vi "Generate Window Name.vi"(10 "Module Name":string, 11 "Item Name":string) -> (3 "Window Name":string)   [LabVIEW 2018, in "MainInterface.lvlib" / "User Interface.lvclass"]
uses:
  User Interface.lvclass
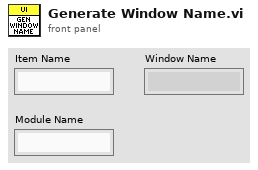
[diagram p1: front panel]
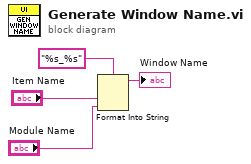
[diagram p0: block diagram]
diagram:
  n1 = Format Into String(format string="%s_%s" ("格式字符串"), "Item Name", "Module Name") -> (resulting string=→"Window Name":string)  [unwired: 2 in, 1 out]
